vi "copy_img_to_gpu.vi"(8 "Error in":errorcluster caption="Error in (no error)", 11 "Hst Src Image (in)":u8[](array[numeric])) -> (0 "Error out":errorcluster, 1 "error_code":i32, 3 "Hst Src Image (out)":u8[](array[numeric]), 4 "Copy to GPU Time (ms)":dbl)   [LabVIEW 2018]
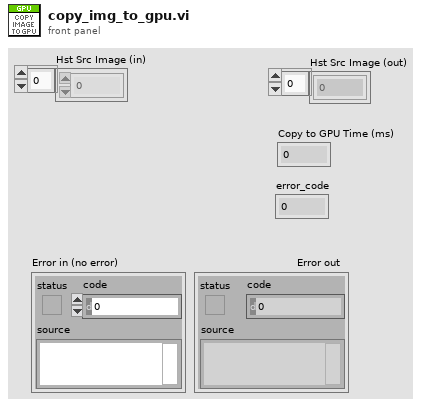
[diagram p1: front panel]
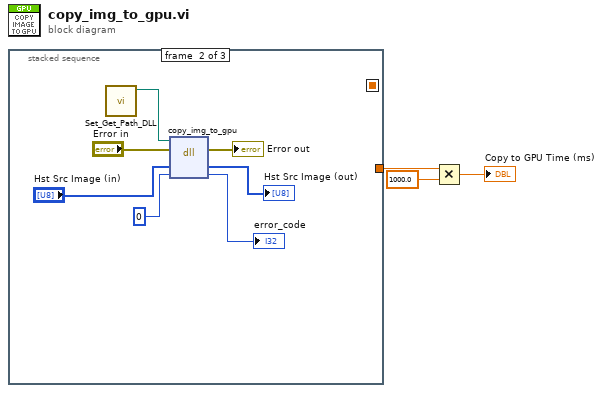
[diagram p0: block diagram]
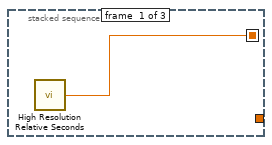
[diagram p2: hidden frame]
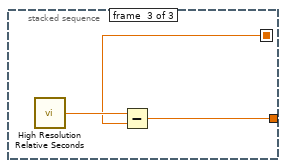
[diagram p3: hidden frame]
diagram:
  n1 = stacked-sequence {
    seq-local: [w4 _ _] -> [_ _ w13]
    tunnel: [_ _ w12] -> w3
    frame #0 {
      n2 = call <vilib>:"High Resolution Relative Seconds.vi"() -> ("relative seconds"=w4:dbl)
    }
    frame #1 {
      n3 = call "Set_Get_Path_DLL.vi"() -> ("path DLL Out"=w5:path)  [unwired: 11 in]
      n4 = dll-call lib="C:/Users/AUTIS/Documents/TFG/Proyecto/Visual Studio/SR_GPU_TOOLKIT_INIT/x64/Release/SR_GPU_TOOLKIT.dll" fn="copy_img_to_gpu"(path in=w5, error in="Error in", "hst_src_image"="Hst Src Image (in)", "error_code"=0) -> (error out=→"Error out":errorcluster, "hst_src_image"=→"Hst Src Image (out)":u8[], "error_code"=→"error_code":i32)  [unwired: 2 in, 1 out]
    }
    frame #2 {
      n5 = call <vilib>:"High Resolution Relative Seconds.vi"() -> ("relative seconds"=w14:dbl)
      n6 = Subtract(x=w14, y=w13) -> (x-y=w12:dbl)
    }
  }
  n7 = Multiply(x=w3, y=1000.0) -> (x*y=→"Copy to GPU Time (ms)":dbl)
